vi "Inst.MOTOR.DoSomething.vi"(8 "error in (no error)":errorcluster, 10 "Data":variant, 11 "Inst.MOTOR in":refnum<class "Inst.MOTOR.lvclass">) -> (0 "error out":errorcluster, 2 "Data out":variant, 3 "Inst.MOTOR out":refnum<class "Inst.MOTOR.lvclass">)   [LabVIEW 2019, in "Inst.MOTOR.lvclass"]
uses:
  Inst.MOTOR.lvclass
  Typedefs/Inst.MOTOR.getAll--Cluster.ctl
  Inst.MOTOR.lvclass/Inst.MOTOR.ctl
  fdab1b40-c942-4d42-9f74-5965e28da6e4.vi
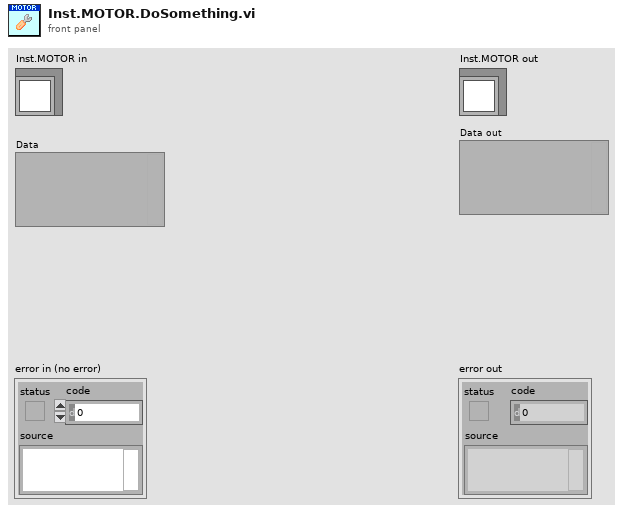
[diagram p1: front panel]
types:
  T1 = typedef "Inst.MOTOR.lvclass/Inst.MOTOR.getAll--Cluster.ctl" = cluster{"Response":string, "Forward":bool, "Stop Motor":bool}
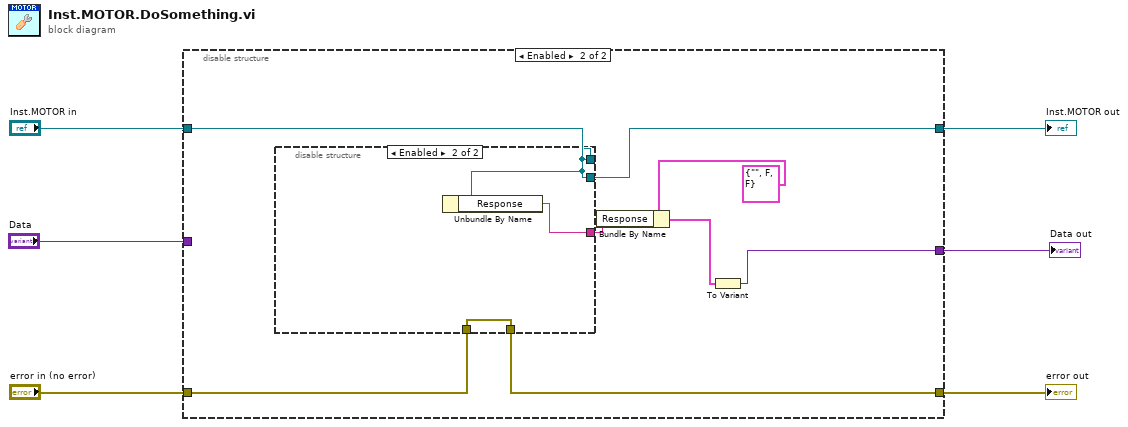
[diagram p0: block diagram]
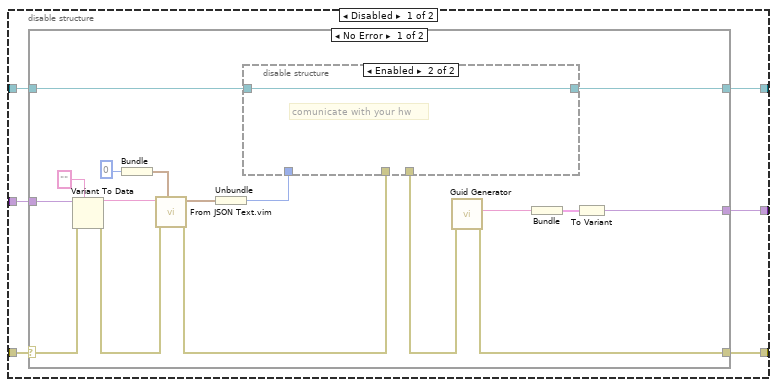
[diagram p2: hidden frame]
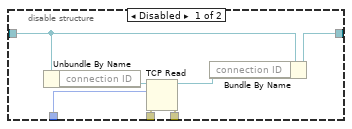
[diagram p3: hidden frame]
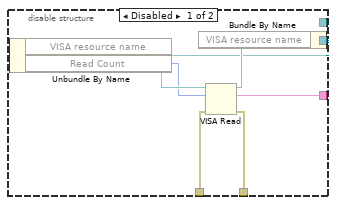
[diagram p5: hidden frame]
diagram:
  n1 = disable-structure shown="Enabled" {
    disable-tunnel: "error in (no error)" -> [w12 w43]
    disable-tunnel: [w11 w42] -> w5
    disable-tunnel: "Inst.MOTOR in" -> [w10 w40]
    disable-tunnel: [w9 w41] -> w3
    disable-tunnel: "Data" -> [w8 _]
    disable-tunnel: [w7 w47] -> w1
    frame Disabled {
      n2 = case shown="No Error" w12 {
        selector: w12 -> [w25 w39]
        tunnel: [w15 w39] -> w11
        tunnel: [w29 w38] -> w9
        tunnel: w10 -> [w28 w38]
        tunnel: w8 -> [w27 _]
        tunnel: [w14 _] -> w7
        frame No Error {
          n3 = Variant To Data(error in=w25, type="", Variant=w27) -> (data=w24:string, error out=w23:errorcluster)
          n4 = Bundle("bytes to read"=0) -> (w21:cluster{"bytes to read":i32})  [unwired: 1 in]
          n5 = call "From JSON Text.vim"("Data Type and Default Value"=w21, "error in (no error)"=w23, "JSON"=w24) -> ("error out"=w22:errorcluster, "Data out"=w20:cluster{"bytes to read":i32})  [unwired: 7 in]
          n6 = Unbundle(w20) -> ("bytes to read"=w19:i32)
          n7 = disable-structure shown="Enabled" {
            disable-tunnel: [w36 w37] -> w29
            disable-tunnel: w28 -> [w35 w37]
            disable-tunnel: w22 -> [w32 _]
            disable-tunnel: w19 -> [w31 _]
            disable-tunnel: [w30 _] -> w16
            frame Disabled {
              n8 = Unbundle By Name(w35) -> ("connection ID"=w34:refnum<k5>)
              n9 = TCP Read(connection ID=w34, bytes to read=w31, error in (no error)=w32) -> (connection ID out=w33:refnum<k5>, error out=w30:errorcluster)  [unwired: 2 in, 1 out]
              n10 = Bundle By Name(cluster=w35, "connection ID"=w33) -> (w36:refnum<class "Inst.MOTOR.lvclass">)
            }
            frame Enabled {
              # "comunicate with your hw"
            }
          }
          n11 = call <vilib>:"Guid Generator.vi"("error in (no error)"=w16) -> ("error out"=w15:errorcluster, "GUID"=w17:string)  [unwired: 9 in]
          n12 = Bundle("GUID"=w17) -> (w13:cluster{"GUID":string})  [unwired: 1 in]
          n13 = To Variant(anything=w13) -> (Variant=w14:variant)
        }
        frame Error {
        }
      }
    }
    frame Enabled {
      n14 = disable-structure shown="Enabled" {
        disable-tunnel: [w54 w56] -> w44
        disable-tunnel: w43 -> [w52 w58]
        disable-tunnel: [w51 w58] -> w42
        disable-tunnel: [w49 w57] -> w41
        disable-tunnel: w40 -> [w48 _]
        disable-tunnel: w40 -> [_ w57]
        frame Disabled {
          n15 = Unbundle By Name(w48) -> ("VISA resource name"=w55:refnum<visa-resource-name>, "Read Count"=w53:u32)
          n16 = VISA Read(VISA resource name=w55, byte count=w53, error in (no error)=w52) -> (VISA resource name out=w50:refnum<visa-resource-name>, read buffer=w54:string, error out=w51:errorcluster)  [unwired: 1 out]
          n17 = Bundle By Name(cluster=w48, "VISA resource name"=w50) -> (w49:refnum<class "Inst.MOTOR.lvclass">)
        }
        frame Enabled {
          n18 = Unbundle By Name(w57) -> ("Response"=w56:string)
        }
      }
      n19 = Bundle By Name(cluster=T1 {"Response"="", "Forward"=FALSE, "Stop Motor"=FALSE} ("getAll"), "Response"=w44) -> (w45:T1)
      n20 = To Variant(anything=w45) -> (Variant=w47:variant)
    }
  }
  "error out" <- w5
  "Inst.MOTOR out" <- w3
  "Data out" <- w1
